vi "DSF.Engine.Interface.Builder.Expected Response.vi"(1 "Command":T3) -> (0 "Response":T1)   [LabVIEW 2017, in "DSF.Engine.lvlib" / "DSF.Engine.Interface.Builder.lvclass"]
uses:
  DSF.Engine.Interface.Builder.lvclass
  DSF.Engine.Interface.Builder.Command Data.ctl
  DSF.Engine.Interface.Builder.Command.ctl
  DSF.Engine.Interface.Builder.Response Data.ctl
  DSF.Engine.Interface.Builder.Response.ctl
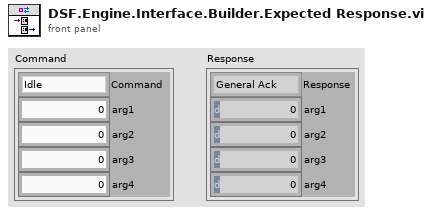
[diagram p1: front panel]
types:
  T1 = typedef "DSF.Engine.lvlib/DSF.Engine.Interface.Builder.lvclass/DSF.Engine.Interface.Builder.Response Data.ctl" = cluster{"Response":T2, "arg1":i32, "arg2":i32, "arg3":i32, "arg4":i32}
  T2 = typedef "DSF.Engine.lvlib/DSF.Engine.Interface.Builder.lvclass/DSF.Engine.Interface.Builder.Response.ctl" = enum8{"General Ack", "Initialize Complete", "Build Complete", "Parse Complete", "Shutdown Ack"}
  T3 = typedef "DSF.Engine.lvlib/DSF.Engine.Interface.Builder.lvclass/DSF.Engine.Interface.Builder.Command Data.ctl" = cluster{"Command":T4, "arg1":i32, "arg2":i32, "arg3":i32, "arg4":i32}
  T4 = typedef "DSF.Engine.lvlib/DSF.Engine.Interface.Builder.lvclass/DSF.Engine.Interface.Builder.Command.ctl" = enum8{"Idle", "Initialize", "Build Buffer", "Parse Buffer", "Shutdown"}
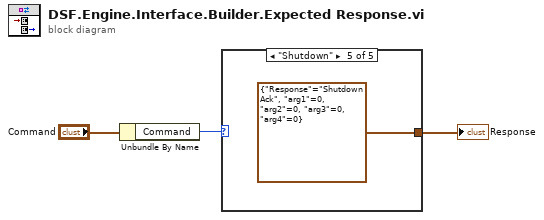
[diagram p0: block diagram]
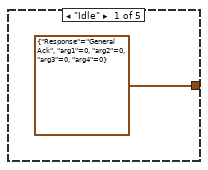
[diagram p2: hidden frame]
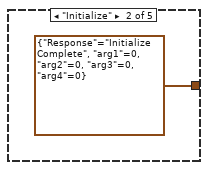
[diagram p3: hidden frame]
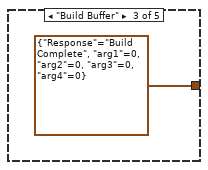
[diagram p4: hidden frame]
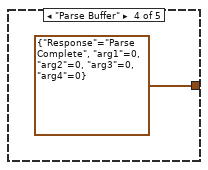
[diagram p5: hidden frame]
diagram:
  n1 = Unbundle By Name("Command") -> ("Command"=w2:T4)
  n2 = case shown="\"Shutdown\"" w2 {
    tunnel: [T1 {"Response"=enum."General Ack", "arg1"=0, "arg2"=0, "arg3"=0, "arg4"=0} ("Response") T1 {"Response"=enum."Initialize Complete", "arg1"=0, "arg2"=0, "arg3"=0, "arg4"=0} ("Response") T1 {"Response"=enum."Build Complete", "arg1"=0, "arg2"=0, "arg3"=0, "arg4"=0} ("Response") T1 {"Response"=enum."Parse Complete", "arg1"=0, "arg2"=0, "arg3"=0, "arg4"=0} ("Response") T1 {"Response"=enum."Shutdown Ack", "arg1"=0, "arg2"=0, "arg3"=0, "arg4"=0} ("Response")] -> w1
    frame "Idle" {
    }
    frame "Initialize" {
    }
    frame "Build Buffer" {
    }
    frame "Parse Buffer" {
    }
    frame "Shutdown" {
    }
  }
  "Response" <- w1
